vi "StopModByName.vi"(8 "ErrorArray In":errorcluster[](array[cluster]), 10 "Module Name":string, 11 "Test.lvclass":refnum<class "Test.lvclass">) -> (0 "ErrorArray Out":errorcluster[](array[cluster]), 1 "Module Stopped":bool, 2 "Module Name out":string, 3 "Test.lvclass":refnum<class "Test.lvclass">, 4 "ModuleRunningNormally?":bool, 5 "Module ID out":i32)   [LabVIEW 2018, in "Test.lvclass"]
doc: "Stops all modules based on the Test Class information (Clone Registration, Module ID, and Module list)."
uses:
  Test.lvclass
  Test.lvclass/Test.ctl
  Accessors/Write CloneReg.vi
  Accessors/Write ModuleIDs.vi
  Accessors/Write ModuleList.vi
  Accessors/Read CloneReg.vi
  Accessors/Read ModuleIDs.vi
  Accessors/Read ModuleList.vi
  <userlib>/NIST/ModuleAdminLib/CloneRegistration/CloneRegistration.lvclass
  <userlib>/NIST/NISTErrorLib/NISTErrorLib.lvlib
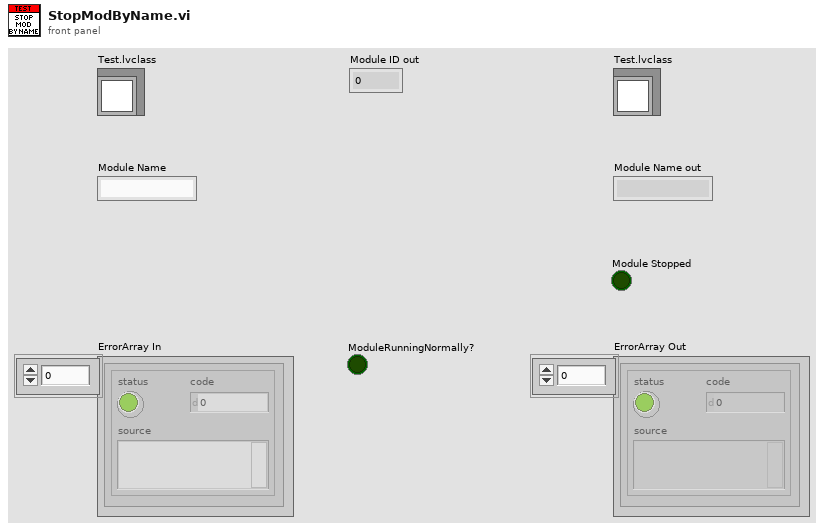
[diagram p1: front panel]
types:
  T1 = enum32{"Bad", "Idle", "Run top level", "Running"}
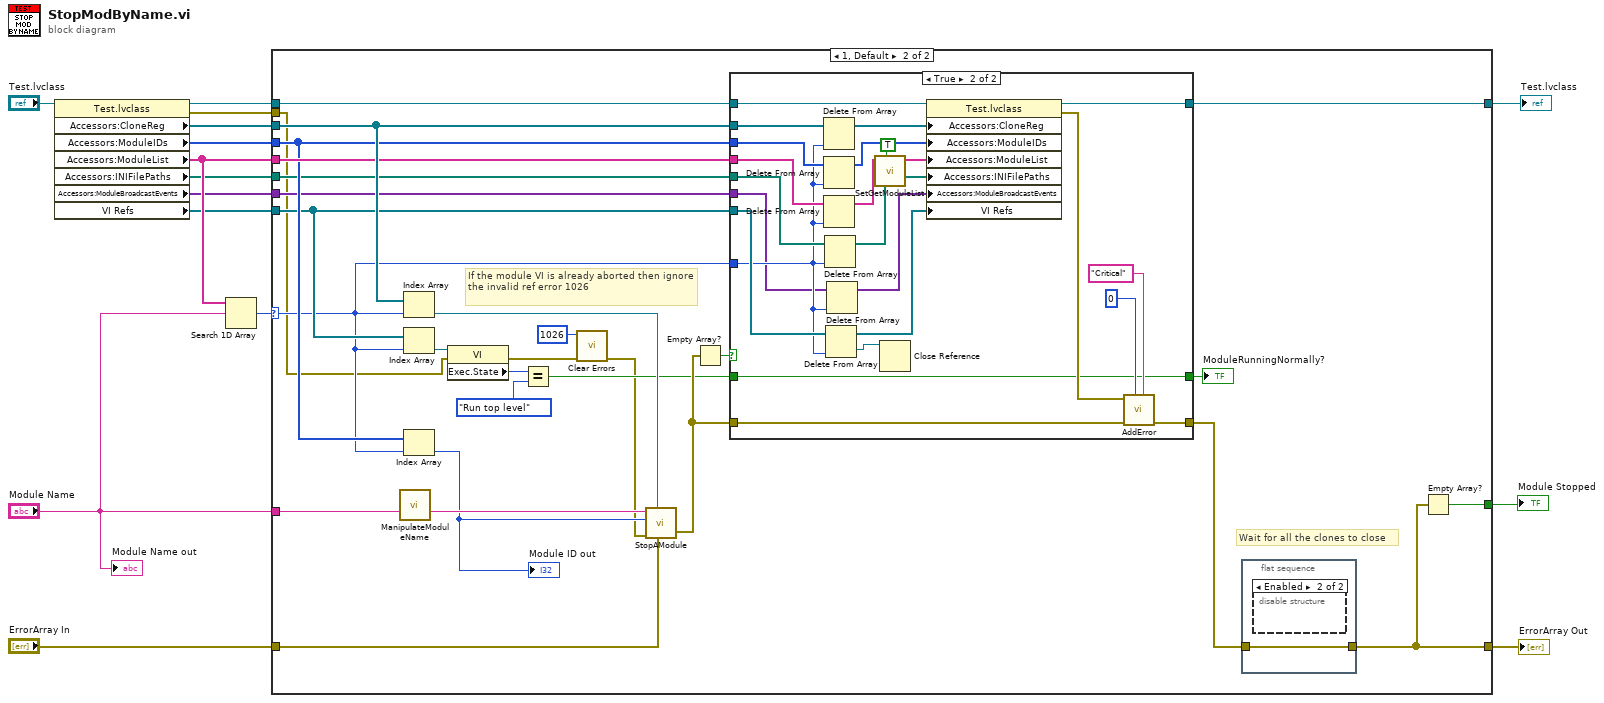
[diagram p0: block diagram]
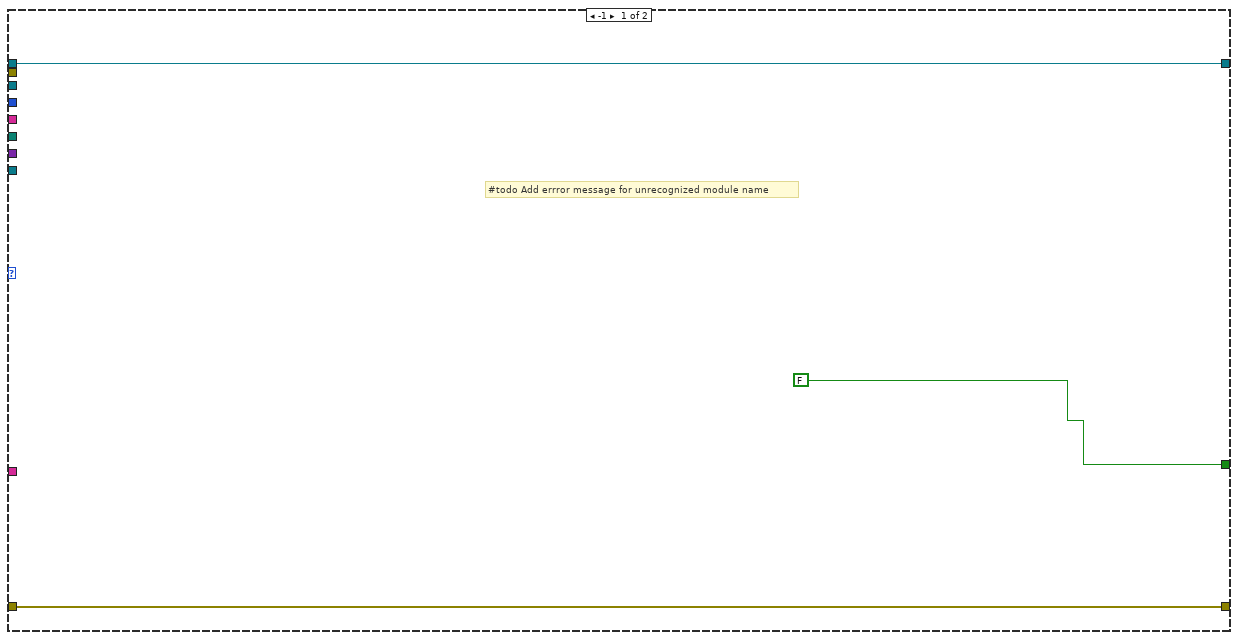
[diagram p2: hidden frame]
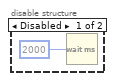
[diagram p3: hidden frame]
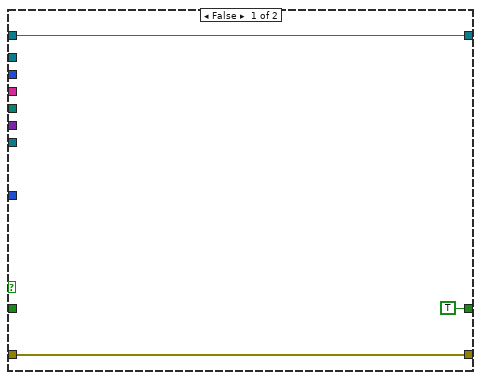
[diagram p4: hidden frame]
diagram:
  n1 = property class="Test.lvclass"(reference="Test.lvclass") -> (reference out=w11:refnum<class "Test.lvclass">, error out=w14:errorcluster, "Accessors:CloneReg"=w10:refnum<data-value>[], "Accessors:ModuleIDs"=w7:i32[], "Accessors:ModuleList"=w9:string[], "Accessors:INIFilePaths"=w3:path[], "Accessors:ModuleBroadcastEvents"=w2:variant[], "VI Refs"=w1:refnum<vi>[])  [unwired: 1 in]
  n2 = Search 1D Array(1D array=w9, element="Module Name") -> (index of element=w6:i32)  [unwired: 1 in]
  n3 = case shown="1, Default" w6 {
    selector: w6 -> [_ w25]
    tunnel: w14 -> [_ w22]
    tunnel: [w17 w36] -> w13
    tunnel: "ErrorArray In" -> [w17 w30]
    tunnel: w11 -> [w18 w45]
    tunnel: w10 -> [_ w43]
    tunnel: w9 -> [_ w40]
    tunnel: "Module Name" -> [_ w39]
    tunnel: w7 -> [_ w38]
    tunnel: [w18 w37] -> w5
    tunnel: [FALSE ("empty?") w35] -> w4
    tunnel: w3 -> [_ w34]
    tunnel: w2 -> [_ w33]
    tunnel: w1 -> [_ w26]
    frame -1 {
      # "#todo Add errror message for unrecognized module name"
    }
    frame 1, Default {
      # "If the module VI is already aborted then ignore the invalid ref error 1026"
      # "Wait for all the clones to close"
      n4 = call "ManipulateModuleName.vi"("ModuleListSingleEntry"=w39) -> ("BeforeMatch:ModuleListSingleEntry"=w46:string)  [unwired: 9 in, 5 out]
      n5 = Index Array(array=w43, index=w25) -> (element=w31:refnum<data-value>)
      n6 = Index Array(array=w26, index=w25) -> (element=w24:refnum<vi>)
      n7 = Index Array(array=w38, index=w25) -> (element=w32:i32)
      "Module ID out" <- w32
      n8 = property class="VI"(reference=w24, error in=w22) -> (error out=w21:errorcluster, "Exec.State"=w28:T1)  [unwired: 1 out]
      n9 = Equal?(x=w28, y=T1."Run top level") -> (x = y?=w23:bool)
      n10 = call <vilib>:"Clear Errors.vi"("error in (no error)"=w21, "specific error code to clear (0: all)"=1026) -> ("error out"=w20:errorcluster)  [unwired: 4 in, 1 out]
      n11 = call "StopAModule.vi"("ErrorArray In"=w30, "Module Clone Reg"=w31, "error in (no error)"=w20, "Module ID"=w32, "Module Name (e.g. Sensor, Digitizer, etc.)"=w46) -> ("ErrorArray Out"=w42:errorcluster[])  [unwired: 6 in]
      n12 = Empty Array?(array=w42) -> (empty?=w44:bool)
      n13 = case shown="True" w44 {
        tunnel: w45 -> [w51 w75]
        tunnel: w43 -> [_ w73]
        tunnel: w38 -> [_ w72]
        tunnel: w40 -> [_ w71]
        tunnel: [w51 w74] -> w37
        tunnel: w25 -> [_ w56]
        tunnel: w42 -> [w50 w65]
        tunnel: [w50 w64] -> w41
        tunnel: w34 -> [_ w62]
        tunnel: w33 -> [_ w53]
        tunnel: w26 -> [_ w57]
        tunnel: [TRUE w54] -> w29
        tunnel: w23 -> [_ w54]
        frame False {
        }
        frame True {
          n14 = Delete From Array(array=w73, index=w56) -> (array with subset deleted=w70:refnum<data-value>[])  [unwired: 1 in, 1 out]
          n15 = Delete From Array(array=w72, index=w56) -> (array with subset deleted=w69:i32[])  [unwired: 1 in, 1 out]
          n16 = Delete From Array(array=w71, index=w56) -> (array with subset deleted=w63:string[])  [unwired: 1 in, 1 out]
          n17 = Delete From Array(array=w62, index=w56) -> (array with subset deleted=w61:path[])  [unwired: 1 in, 1 out]
          n18 = Delete From Array(array=w57, index=w56) -> (deleted portion=w52:refnum<vi>, array with subset deleted=w55:refnum<vi>[])  [unwired: 1 in]
          n19 = Delete From Array(array=w53, index=w56) -> (array with subset deleted=w60:variant[])  [unwired: 1 in, 1 out]
          n20 = call "SetGetModuleList.vi"("Set? (F)"=TRUE, "ModuleList"=w63) -> ("ModuleList"=w59:string[])  [unwired: 9 in]
          n21 = Close Reference(reference=w52) -> ()  [unwired: 1 in, 1 out]
          n22 = property class="Test.lvclass"(reference=w75, "Accessors:CloneReg"=w70, "Accessors:ModuleIDs"=w69, "Accessors:ModuleList"=w59, "Accessors:INIFilePaths"=w61, "Accessors:ModuleBroadcastEvents"=w60, "VI Refs"=w55) -> (reference out=w74:refnum<class "Test.lvclass">, error out=w66:errorcluster)  [unwired: 1 in]
          n23 = call <userlib>:"AddError.vi"("Severity"="Critical", "Priority"=u8 0, "ErrorArray In"=w65, "error in (no error)"=w66) -> ("ErrorArray Out"=w64:errorcluster[])  [unwired: 6 in, 1 out]
        }
      }
      "ModuleRunningNormally?" <- w29
      n24 = flat-sequence {
        tunnel: [w47] -> w36
        tunnel: w41 -> [w47]
        frame #0 {
          n25 = disable-structure shown="Enabled" {
            frame Disabled {
              n26 = Wait (ms)(milliseconds to wait=u32 2000) -> ()  [unwired: 1 out]
            }
            frame Enabled {
            }
          }
        }
      }
      n27 = Empty Array?(array=w36) -> (empty?=w35:bool)
    }
  }
  "ErrorArray Out" <- w13
  "Test.lvclass" <- w5
  "Module Stopped" <- w4
  "Module Name out" <- "Module Name"
